vi "Show TortoiseGit Log.vi"(8 "error in":errorcluster, 10 "/path value":string, 11 "Working Directory":path) -> (0 "error out":errorcluster)   [LabVIEW 2018, in "TortoiseGit Show Log.lvlib"]
doc: "Calls command prompt to launch TortoiseGit log at either the repo or for a specific folder path/VI."
uses:
  TortoiseGit Show Log.lvlib
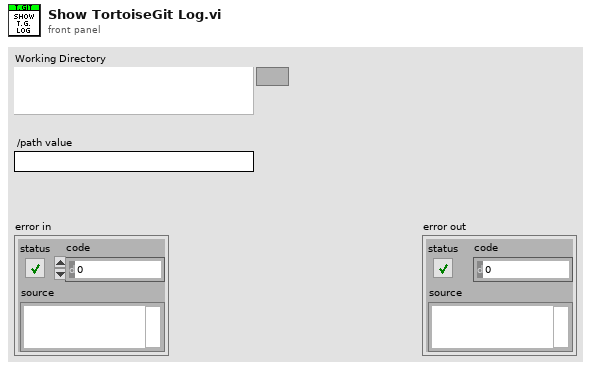
[diagram p1: front panel]
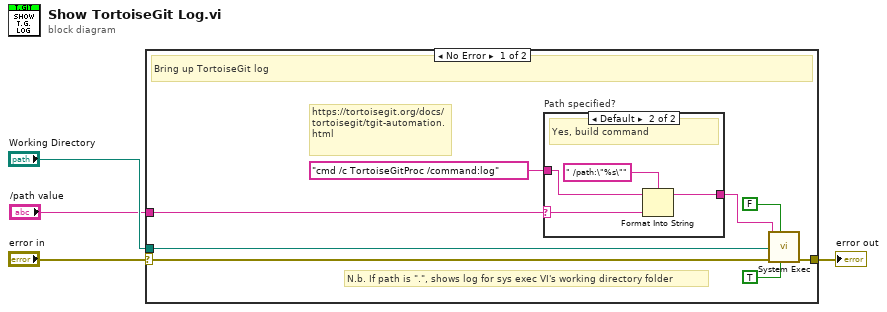
[diagram p0: block diagram]
diagram:
  n1 = case shown="No Error" "error in" {
    selector: "error in" -> [w11 w18]
    tunnel: [w12 w18] -> w1
    tunnel: "Working Directory" -> [w10 _]
    tunnel: "/path value" -> [w9 _]
    frame No Error {
      # "N.b. If path is \".\", shows log for sys exec VI's working directory folder"
      # "https://tortoisegit.org/docs/tortoisegit/tgit-automation.html"
      # "Bring up TortoiseGit log"
      n2 = case "Path specified?" shown="Default" w9 {
        selector: w9 -> [_ w16]
        tunnel: "cmd /c TortoiseGitProc /command:log" ("format string") -> [w13 w14]
        tunnel: [w13 w15] -> w7
        frame "" {
          # "No --> Don't append path  to command (shows repo)"
        }
        frame Default {
          # "Yes, build command"
          n3 = Format Into String(format string=" /path:\"%s\"" ("false string"), initial string=w14, w16) -> (resulting string=w15:string)  [unwired: 1 in, 1 out]
        }
      }
      n4 = call <vilib>:"System Exec.vi"("run minimized? (F)"=TRUE, "wait until completion? (T)"=FALSE, "error in (no error)"=w11, "working directory"=w10, "command line"=w7) -> ("error out"=w12:errorcluster)  [unwired: 3 in, 3 out]
    }
    frame Error {
      # "Don't bring up log, pass out error"
    }
  }
  "error out" <- w1
